vi "disdrometer_PreventUserStrings.vi"(11 "UserCommand":string) -> (1 "UserMessage":string, 2 "Filtered?":bool, 3 "Filtered Command":string)   [LabVIEW 2018]
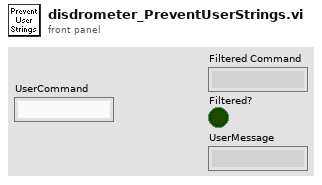
[diagram p1: front panel]
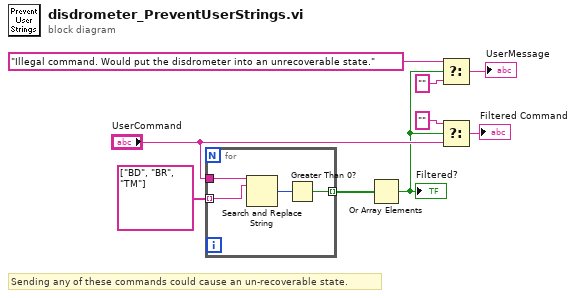
[diagram p0: block diagram]
diagram:
  # "Sending any of these commands could cause an un-recoverable state."
  n1 = for {
    tunnel: string[] ["BD", "BR", "TM"] ("search string") -> [w13] mode=indexing
    tunnel: "UserCommand" -> [w12]
    tunnel: [w10] -> w8 mode=indexing
    n2 = Search and Replace String(input string=w12, search string=w13) -> (number of replacements=w11:i32)  [unwired: 6 in, 3 out]
    n3 = Greater Than 0?(x=w11) -> (x > 0?=w10:bool)
  }
  n4 = Or Array Elements(Boolean array=w8) -> (logical OR=w3:bool)
  "Filtered?" <- w3
  n5 = Select(t="Illegal command. Would put the disdrometer into an unrecoverable state.", s=w3, f="" ("t")) -> (s? t:f=→"UserMessage":string)
  n6 = Select(t="", s=w3, f="UserCommand") -> (s? t:f=→"Filtered Command":string)
